vi "Send Configure Burst Count [BST].vi"(7 "Message Priority (Normal)":T1=enum."Normal", 8 "error in (no error)":errorcluster, 9 "burst count (1)":i32=1, 10 "Channel Name (\"\")":string="CHANNEL1" caption="channel name (\"CHANNEL1\")", 11 "Message Enqueuer":refnum<class "Message Enqueuer.lvclass">) -> (0 "error out":errorcluster, 3 "Message Enqueuer out":refnum<class "Message Enqueuer.lvclass">)   [LabVIEW 2016, in "CS++Fgen.lvlib" / "Configure Burst Count [BST] Msg.lvclass"]
doc: "Sends the <B>CS++Fgen.lvlib:Configure Burst Count [BST] Msg.lvclass</B> message.\n\n<B>CS++Fgen.lvlib:CS++Fgen.lvclass:Configure Burst Count [BST].vi</B> Description:\n\nThis VI configures the burst count. When the function generator receives a trigger while in the Burst operation mode, it generates the number of waveform cycles you specify in the Count control.\n\nNotes:\n\n(1) This VI is part of the IviFgenBurst [BST] extension group."
uses:
  Configure Burst Count [BST] Msg.lvclass
  <vilib>/ActorFramework/Message Enqueuer/Message Enqueuer.lvclass
  <vilib>/ActorFramework/Message Enqueuer/Message Priority.ctl
  C:/Program Files (x86)/National Instruments/LabVIEW 2016/vi.lib/ActorFramework/Message/Message.lvclass
  Configure Burst Count [BST] Msg.lvclass/Configure Burst Count [BST] Msg.ctl
  <vilib>/ActorFramework/Message Enqueuer/Message Enqueuer.lvclass/Message Enqueuer.ctl
  <vilib>/ActorFramework/Message Priority Queue/Priority Enqueue.vi
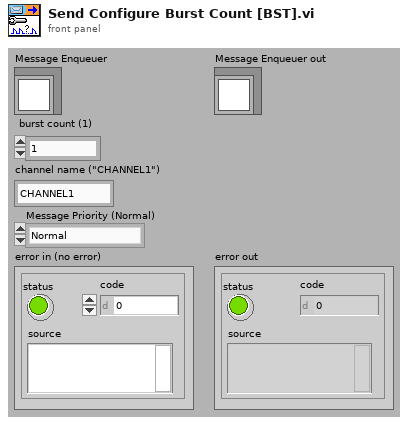
[diagram p1: front panel]
types:
  T1 = typedef "Actor Framework.lvlib/Message Enqueuer.lvclass/Message Priority.ctl" = enum16{"Low", "Normal", "High"}
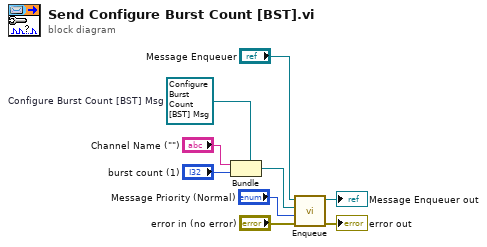
[diagram p0: block diagram]
diagram:
  w3 = refnum<class "Configure Burst Count [BST] Msg.lvclass"> refnum  # Configure Burst Count [BST] Msg
  n1 = Bundle(cluster=w3, "Channel Name (\"\")", "burst count (1)") -> (w6:refnum<class "Configure Burst Count [BST] Msg.lvclass">)
  n2 = call <vilib>:"Enqueue.vi"("error in (no error)"="error in (no error)", "Message Priority (Normal)"="Message Priority (Normal)", "Message"=w6, "Message Enqueuer in"="Message Enqueuer") -> ("error out"=→"error out":errorcluster, "Message Enqueuer out"=→"Message Enqueuer out":refnum<class "Message Enqueuer.lvclass">)  [unwired: 6 in]
